vi "Split output descriptions.vi"(11 "output descriptions combined":string[][](array[string])) -> (2 "output descriptions 2":string[][](array[string]), 3 "output descriptions":string[][](array[string]))   [LabVIEW 2012]
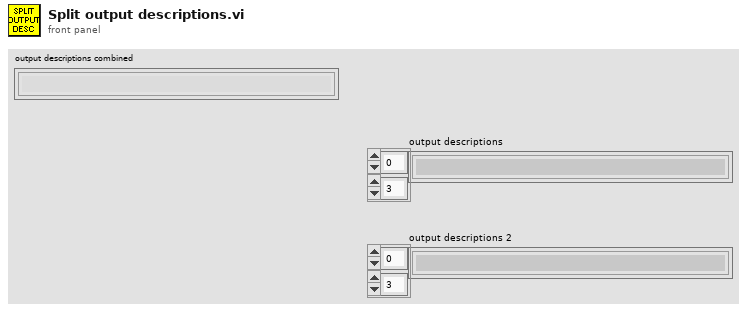
[diagram p1: front panel]
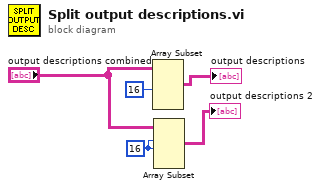
[diagram p0: block diagram]
diagram:
  w3 = 16 ("length")
  n1 = Array Subset(array="output descriptions combined", length (row)=16 ("length")) -> (→"output descriptions":string[][])  [unwired: 3 in]
  n2 = Array Subset(array="output descriptions combined", index (row)=w3, length (row)=w3) -> (→"output descriptions 2":string[][])  [unwired: 2 in]
